vi "SHA_calc_appendsU32.vi"(11 "String length":i32) -> (2 "Append":u8[](array[numeric]), 3 "Number of chunks":i32)   [LabVIEW 2011, in "i3-external-encryption.lvlib"]
doc: "Calculates the appendices for the last chunks (32-bit).\n\n(c) Ton Plomp, 2011\nTHIS SOFTWARE IS PROVIDED AS IS, AND ANY WARRANTY IS REJECTED"
uses:
  i3-external-encryption.lvlib
panel:
  out "x+y":i32
  out "length":i32
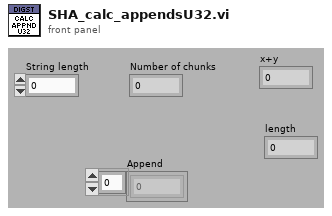
[diagram p1: front panel]
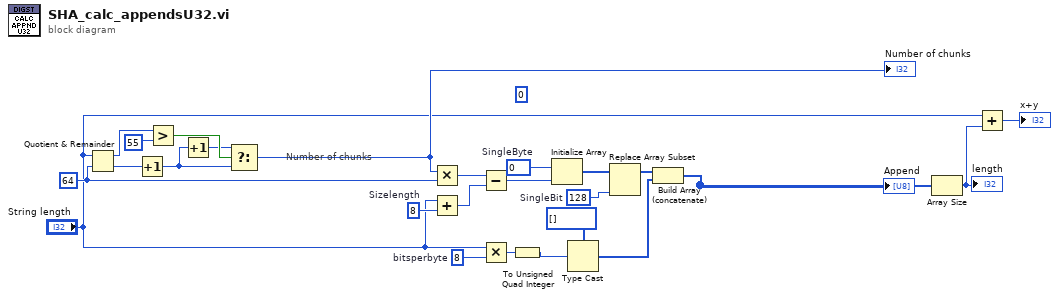
[diagram p0: block diagram]
diagram:
  (unwired) 0
  w16 = 8  # Sizelength
  w9 = u8 0  # SingleByte
  w8 = 8  # bitsperbyte
  w14 = 64 ("y")
  w11 = u8 128  # SingleBit
  # "Number of chunks"
  n1 = Quotient & Remainder(x="String length", y=w14) -> (x-y*floor(x/y)=w21:i32, floor(x/y)=w18:i32)
  n2 = Increment(x=w18) -> (x+1=w23:i32)
  n3 = Greater?(x=w21, y=55) -> (0:w25:bool)
  n4 = Increment(x=w23) -> (x+1=w22:i32)
  n5 = Select(t=w22, s=w25, f=w23) -> (s? t:f=w24:i32)
  "Number of chunks" <- w24
  n6 = Multiply(x=w24, y=w14) -> (x*y=w19:i32)
  n7 = Add(x="String length", y=w16) -> (x+y=w15:i32)
  n8 = Subtract(x=w19, y=w15) -> (x-y=w17:i32)
  n9 = Multiply(x="String length", y=w8) -> (x*y=w10:i32)
  n10 = To Unsigned Quad Integer(1:w10) -> (0:w2:u64)
  n11 = Initialize Array(w9, w17) -> (w12:u8[])
  n12 = Type Cast(type=u8[] [], x=w2) -> (*(type *) &x=w1:u8[])
  n13 = Replace Array Subset(array=w12, new element=w11) -> (w13:u8[])  [unwired: 1 in]
  n14 = Build Array (concatenate)(w13, w1) -> (w7:u8[])
  "Append" <- w7
  n15 = Array Size(array=w7) -> (size(s)=w5:i32)
  "length" <- w5
  n16 = Add(x="String length", y=w5) -> (x+y=→"x+y":i32)
